vi "Array Average.vi"() -> ()   [LabVIEW 2024]
panel:
  out "Array average":dbl
  in  "Input array":dbl[](array[numeric])
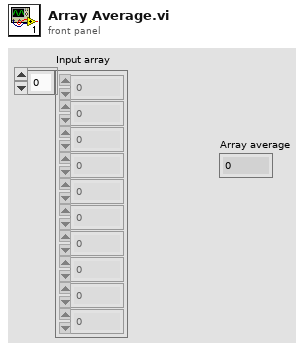
[diagram p1: front panel]
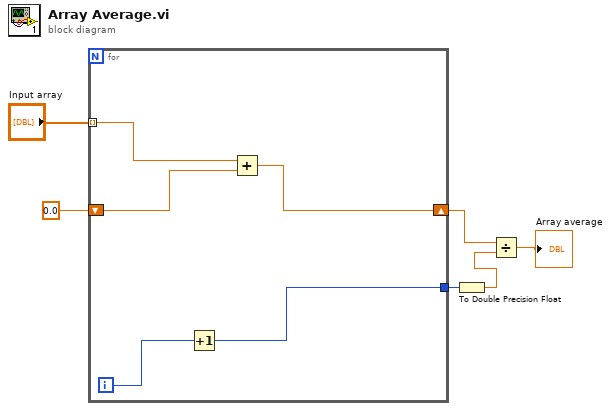
[diagram p0: block diagram]
diagram:
  n1 = for {
    tunnel: "Input array" -> [w10] mode=indexing
    shift-right: [w11] -> w1
    shift-left: 0.0 -> [w9]
    tunnel: [w7] -> w4
    i -> [w8]
    n2 = Increment(x=w8) -> (x+1=w7:i32)
    n3 = Add(x=w10, y=w9) -> (x+y=w11:dbl)
  }
  n4 = To Double Precision Float(number=w4) -> (double precision float=w2:dbl)
  n5 = Divide(x=w1, y=w2) -> (x/y=→"Array average":dbl)
